vi "sub_calXYZcoordinates.vi"(8 "Vertical Correction":dbl, 9 "distance (meter)":dbl, 10 "vertical (degree)":dbl, 11 "azimuth (degree)":dbl) -> (0 "R (meter)":dbl, 1 "Z (meter)":dbl, 2 "Y (meter)":dbl, 3 "X (meter)":dbl)   [LabVIEW 2020]
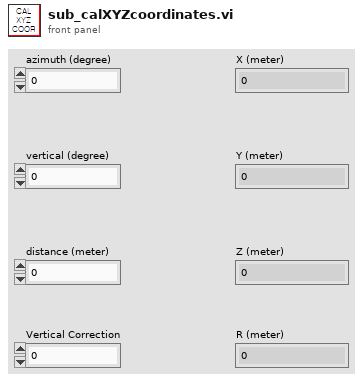
[diagram p1: front panel]
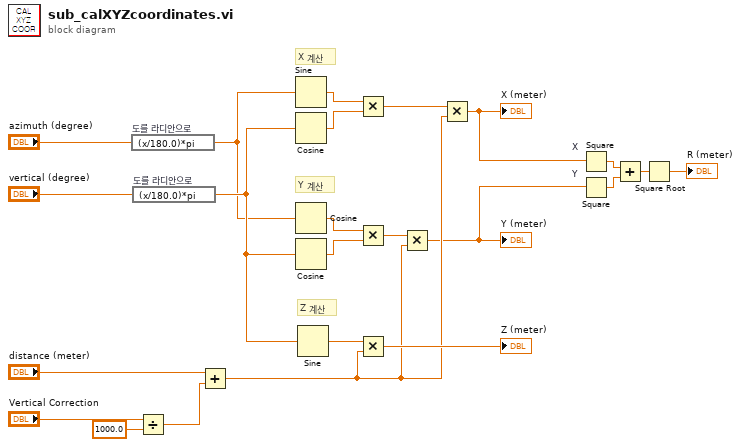
[diagram p0: block diagram]
diagram:
  # "Z 계산"
  # "Y 계산"
  # "X 계산"
  n1 = expression code="(x/180.0)*pi" "도를 라디안으로"("azimuth (degree)") -> (w14:dbl)
  n2 = expression code="(x/180.0)*pi" "도를 라디안으로"("vertical (degree)") -> (w15:dbl)
  n3 = Divide(x="Vertical Correction", y=1000.0) -> (x/y=w7:dbl)
  n4 = Add(x="distance (meter)", y=w7) -> (x+y=w10:dbl)
  n5 = Sine(x=w14) -> (sin(x)=w16:dbl)
  n6 = Cosine(x=w15) -> (cos(x)=w17:dbl)
  n7 = Cosine(x=w14) -> (cos(x)=w18:dbl)
  n8 = Cosine(x=w15) -> (cos(x)=w19:dbl)
  n9 = Sine(x=w15) -> (sin(x)=w20:dbl)
  n10 = Multiply(x=w16, y=w17) -> (x*y=w21:dbl)
  n11 = Multiply(x=w18, y=w19) -> (x*y=w22:dbl)
  n12 = Multiply(x=w20, y=w10) -> (x*y=→"Z (meter)":dbl)
  n13 = Multiply(x=w22, y=w10) -> (x*y=w2:dbl)
  "Y (meter)" <- w2
  n14 = Multiply(x=w21, y=w10) -> (x*y=w3:dbl)
  "X (meter)" <- w3
  n15 = Square "X"(x=w3) -> (x^2=w6:dbl)
  n16 = Square "Y"(x=w2) -> (x^2=w5:dbl)
  n17 = Add(x=w6, y=w5) -> (x+y=w4:dbl)
  n18 = Square Root(x=w4) -> (sqrt(x)=→"R (meter)":dbl)
